vi "删除解压替换.vi"() -> (0 "操作失败?":bool=TRUE)   [LabVIEW 2017]
uses:
  <vilib>/zip/NI_Unzip.lvlib
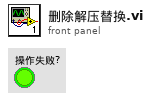
[diagram p1: front panel]
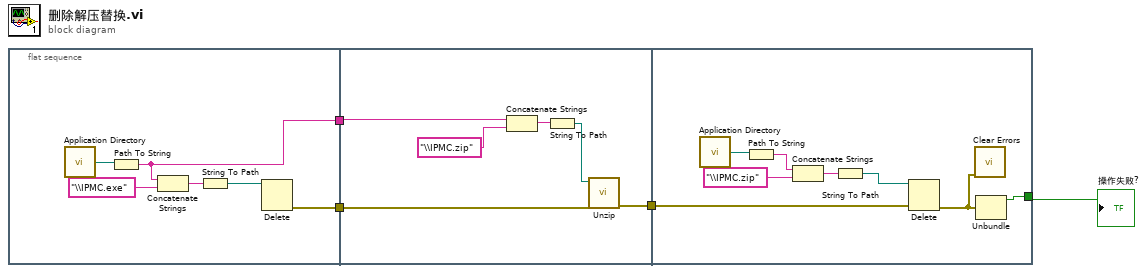
[diagram p0: block diagram]
diagram:
  n1 = flat-sequence {
    tunnel: [w6] -> w4
    tunnel: [w5] -> w3
    tunnel: w4 -> [w13]
    tunnel: w3 -> [w12]
    tunnel: [w11] -> w2
    tunnel: w2 -> [w19]
    tunnel: [w17] -> w1
    frame #0 {
      n2 = call <vilib>:"Application Directory.vi"() -> ("Application Directory"=w9:path)
      n3 = Path To String(path=w9) -> (string=w6:string)
      n4 = Concatenate Strings(w6, "\\IPMC.exe") -> (w8:string)
      n5 = String To Path(string=w8) -> (path=w7:path)
      n6 = Delete(path (use dialog)=w7) -> (error out=w5:errorcluster)  [unwired: 4 in, 2 out]
    }
    frame #1 {
      n7 = Concatenate Strings(w13, "\\IPMC.zip") -> (w15:string)
      n8 = String To Path(string=w15) -> (path=w16:path)
      n9 = call <vilib>:"Unzip.vi"("error in (no error)"=w12, "Zip file"=w16) -> ("error out"=w11:errorcluster)  [unwired: 7 in, 2 out]
    }
    frame #2 {
      n10 = call <vilib>:"Application Directory.vi"() -> ("Application Directory"=w23:path)
      n11 = Path To String(path=w23) -> (string=w20:string)
      n12 = Concatenate Strings(w20, "\\IPMC.zip") -> (w22:string)
      n13 = String To Path(string=w22) -> (path=w21:path)
      n14 = Delete(path (use dialog)=w21, error in=w19) -> (error out=w18:errorcluster)  [unwired: 3 in, 2 out]
      n15 = call <vilib>:"Clear Errors.vi"("error in (no error)"=w18) -> ()  [unwired: 5 in, 2 out]
      n16 = Unbundle(w18) -> ("status"=w17:bool)  [unwired: 2 out]
    }
  }
  "操作失败?" <- w1
